vi "Main Single Channel Only.vi"() -> ()   [LabVIEW 2017]
uses:
  Controls/Timing Controls.ctl
  Controls/File Controls.ctl
  Controls/DAQ State.ctl
  <vilib>/DAQmx/write.llb/DAQmx Write (Analog 1D DBL NChan 1Samp).vi
  <vilib>/DAQmx/configure/timing.llb/DAQmx Timing (Sample Clock).vi
  <vilib>/DAQmx/miscellaneous.llb/DAQmx Fill In Error Info.vi
panel:
  in  "Trigger Channel (Find Using NI Max)":tag="Dev1/ai16"
  in  "Differential Value":dbl format="%#_13g"
  in  "Lower Limit":dbl=-0.85
  in  "Upper Limit":dbl=-0.75
  out "Differential":cluster{dbl[], dbl[]}[](graph)=[{[0.0, 1.0], [0.0029010882279960626, 0.00862868344710327]}, {[-1.0, 2.0], [-0.75, -0.75]}, {[-1.0, 2.0], [-0.85, -0.85]}]
  out "Saving?":bool
  out "Zero Values Dev1":dbl[](array[numeric])
  in  "Save":bool
  in  "File Control":T1={"File Path"=path "C:/Users/Force PC/Documents/Acquisition Data", "File Name"=""}
  out "Trigger":dynamicdata(graph)=[{"t0"=timestamp(3616576961.7901273 s since 1904-01-01), "dt"=0.001, "Y"=[2.8935987566836108, 2.892940411376444, 2.8932695840305964, 2.8932695840305964, 2.8932695840305964, 2.8932695840305964, 2.8934341703572457, 2.8935987566836108, 2.8935987566836108, 2.893763343009691, 2.8934341703572457, 2.8940925156609985, 2.8940925156609985, 2.8942571019862253, 2.8940925156609985, 2.8935987566836108, 2.893927929335487, 2.893763343009691, 2.893763343009691, 2.8934341703572457, 2.8932695840305964, 2.8932695840305964, 2.8931049977036625, 2.8934341703572457, 2.8931049977036625, 2.8932695840305964, 2.8931049977036625, 2.8935987566836108, 2.893927929335487, 2.893927929335487, 2.893763343009691, 2.8942571019862253, 2.8942571019862253, 2.8940925156609985, 2.893927929335487, 2.893927929335487, 2.893763343009691, 2.893763343009691, 2.8935987566836108, 2.8932695840305964, 2.8934341703572457, 2.892775825048941, 2.8931049977036625, 2.892940411376444, 2.8931049977036625, 2.8934341703572457, 2.8934341703572457, 2.893763343009691, 2.893763343009691, 2.893927929335487, 2.893763343009691, 2.894421688311168, 2.8942571019862253, 2.894421688311168, 2.8940925156609985, 2.893927929335487, 2.894421688311168, 2.894421688311168, 2.893763343009691, 2.8934341703572457, 2.893927929335487, 2.892940411376444, 2.8935987566836108, 2.8931049977036625, 2.8934341703572457, 2.8935987566836108, 2.8935987566836108, 2.893763343009691, 2.893763343009691, 2.8942571019862253, 2.893927929335487, 2.894421688311168, 2.8947508609601993, 2.894421688311168, 2.8940925156609985, 2.8940925156609985, 2.8942571019862253, 2.8940925156609985, 2.893763343009691, 2.8935987566836108, 2.8934341703572457, 2.8931049977036625, 2.892940411376444, 2.8931049977036625, 2.8932695840305964, 2.8931049977036625, 2.8932695840305964, 2.8935987566836108, 2.8935987566836108, 2.8942571019862253, 2.893927929335487, 2.894421688311168, 2.893927929335487, 2.894586274635826, 2.893927929335487, 2.8942571019862253, 2.893927929335487, 2.8940925156609985, 2.893763343009691, 2.8932695840305964], "attributes"=variant("NI_ChannelName"=variant(string "Trigger"), "NI_UnitDescription"=variant(string "Volts"))}]
  out "Dev1":dynamicdata(graph)=[{"t0"=timestamp(3616576961.790079 s since 1904-01-01), "dt"=0.001, "Y"=[0.004713341620051992, 0.0045485913126213084, 0.005042842234350253, 0.0052075925412182755, 0.004219090697197281, 0.0038895900810222983, 0.004219090697197281, 0.0043838410050032195, 0.0038895900810222983, 0.0037248397726536986, 0.004713341620051992, 0.0045485913126213084, 0.0045485913126213084, 0.004054340389203492, 0.0038895900810222983, 0.004713341620051992, 0.004713341620051992, 0.003395339155353394, 0.004878091927295269, 0.004219090697197281, 0.0038895900810222983, 0.003395339155353394, 0.004219090697197281, 0.004713341620051992, 0.0030658385373025787, 0.003395339155353394, 0.0038895900810222983, 0.003395339155353394, 0.0038895900810222983, 0.003230588846421689, 0.003560089464097249, 0.003230588846421689, 0.002571587608819481, 0.003230588846421689, 0.0029010882279960626, 0.0037248397726536986, 0.0030658385373025787, 0.0037248397726536986, 0.0037248397726536986, 0.003560089464097249, 0.003230588846421689, 0.0037248397726536986, 0.003230588846421689, 0.0027363379185016967, 0.0027363379185016967, 0.002571587608819481, 0.003230588846421689, 0.003560089464097249, 0.0037248397726536986, 0.0029010882279960626, 0.0037248397726536986, 0.003395339155353394, 0.003560089464097249, 0.003395339155353394, 0.0038895900810222983, 0.0029010882279960626, 0.003230588846421689, 0.0030658385373025787, 0.0027363379185016967, 0.003395339155353394, 0.0030658385373025787, 0.004054340389203492, 0.003560089464097249, 0.0037248397726536986, 0.0029010882279960626, 0.003230588846421689, 0.002571587608819481, 0.0027363379185016967, 0.0030658385373025787, 0.004054340389203492, 0.0027363379185016967, 0.00240683729894986, 0.002571587608819481, 0.0019125863682161182, 0.0027363379185016967, 0.0029010882279960626, 0.0030658385373025787, 0.0027363379185016967, 0.0030658385373025787, 0.0029010882279960626, 0.00240683729894986, 0.0030658385373025787, 0.0027363379185016967, 0.00240683729894986, 0.002571587608819481, 0.0030658385373025787, 0.003230588846421689, 0.002571587608819481, 0.002242086988892833, 0.003230588846421689, 0.002242086988892833, 0.002242086988892833, 0.0030658385373025787, 0.002571587608819481, 0.003230588846421689, 0.002571587608819481, 0.00240683729894986, 0.004054340389203492, 0.0029010882279960626, 0.0029010882279960626], "attributes"=variant("NI_ChannelName"=variant(string "Dev1_Ch3"), "NI_UnitDescription"=variant(string "Volts"))}]
  in  "Zero Dev1":bool caption="Zero"
  in  "Timing":T2={"Sampling Rate (Hz)"=1000.0, "Display Rate (Hz)"=100.0, "Sampling Mode"=10123} {"Sampling Mode" items=["Finite Samples"=10178, "Continuous Samples"=10123, "Hardware Timed Single Point"=12522]; "Sampling Rate (Hz)" format="%0.2f"}
  in  "Run":bool
  out "DAQ \nConnected?":bool
  in  "stop":bool
  # "You shouldn't need to change this,\nunless the trigger is not showing up.\nUse NI MAX -> Test Panels\nWill be between ai16 and ai31\nThis must be set before the program\nruns"
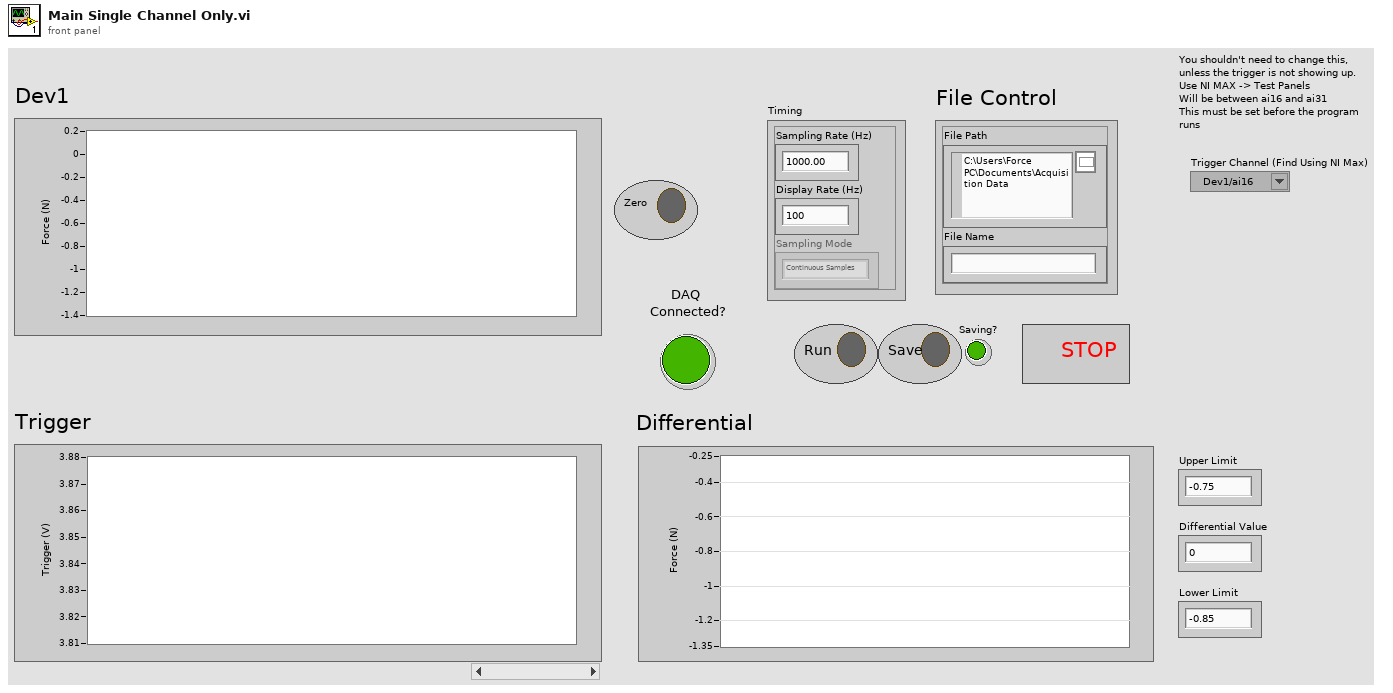
[diagram p1: front panel]
types:
  T1 = typedef "File Controls.ctl" = cluster{"File Path":path, "File Name":string}
  T2 = typedef "Timing Controls.ctl" = cluster{"Sampling Rate (Hz)":dbl, "Display Rate (Hz)":dbl, "Sampling Mode":i32}
  T3 = cluster{"Waveform Array":waveform(dbl)[][], bool}
  T4 = typedef "DAQ State.ctl" = enum16{"Init", "Wait", "Update Timing", "Zero Dev1", "Zero Dev2", "Start Task", "Read", "Stop Task", "Display Data", "Write to File", "Error Handling", "Shutdown"}
  T5 = enum8{"Enabled", "Disabled", "Disabled and Grayed Out"}
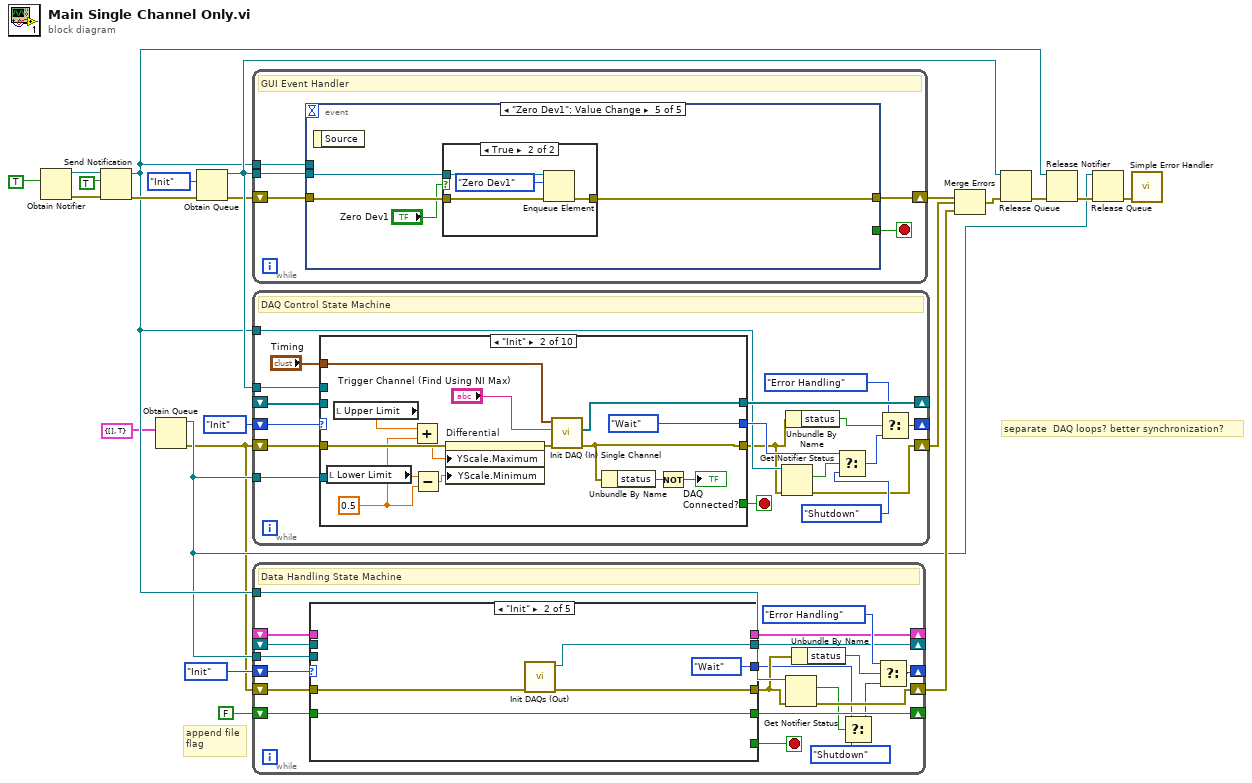
[diagram p0: block diagram]
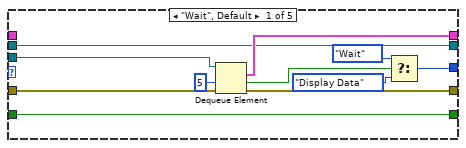
[diagram p2: hidden frame]
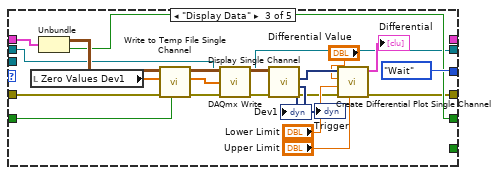
[diagram p3: hidden frame]
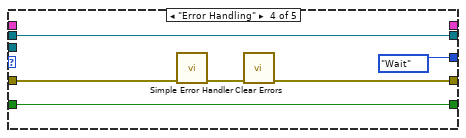
[diagram p4: hidden frame]
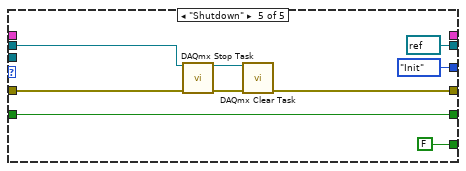
[diagram p5: hidden frame]
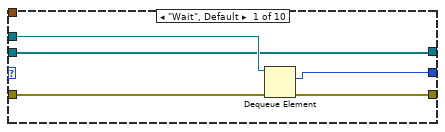
[diagram p6: hidden frame]
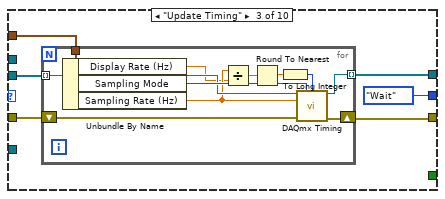
[diagram p7: hidden frame]
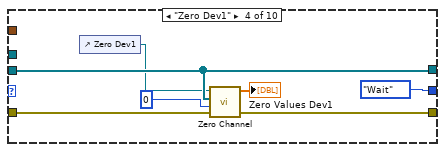
[diagram p8: hidden frame]
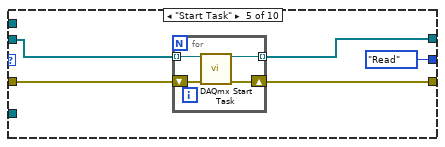
[diagram p9: hidden frame]
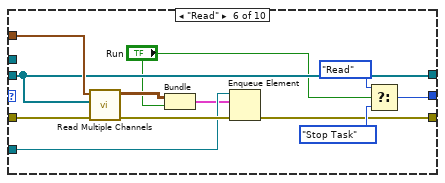
[diagram p10: hidden frame]
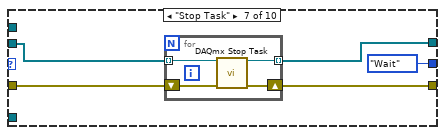
[diagram p11: hidden frame]
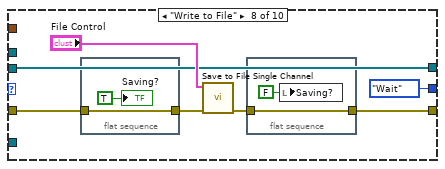
[diagram p12: hidden frame]
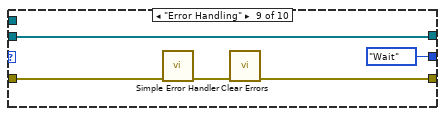
[diagram p13: hidden frame]
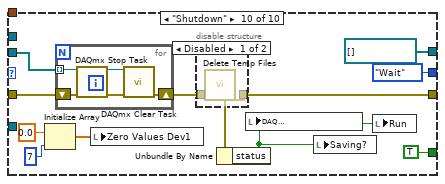
[diagram p14: hidden frame]
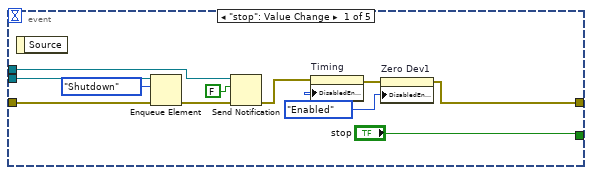
[diagram p16: hidden frame]
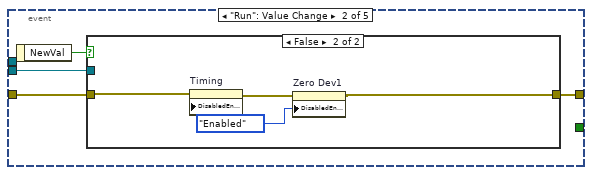
[diagram p17: hidden frame]
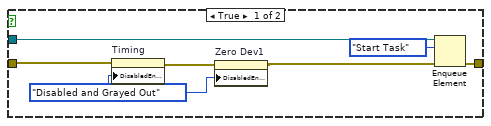
[diagram p18: hidden frame]
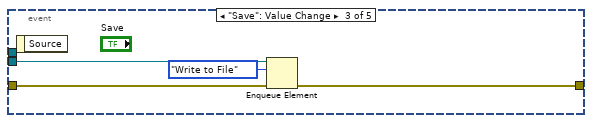
[diagram p19: hidden frame]
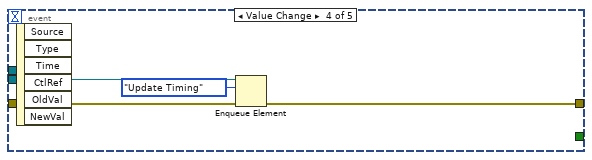
[diagram p20: hidden frame]
diagram:
  # "append file\nflag"
  # "separate  DAQ loops? better synchronization?"
  n1 = Obtain Notifier(notification data type=TRUE) -> (notifier out=w13:refnum<notifier>, error out=w12:errorcluster)  [unwired: 3 in, 1 out]
  n2 = Send Notification(notification=TRUE, notifier=w13, error in (no error)=w12) -> (notifier out=w9:refnum<notifier>, error out=w11:errorcluster)
  n3 = Obtain Queue(element data type=T3 {"Waveform Array"=[], TRUE}) -> (queue out=w6:refnum<queue>, error out=w2:errorcluster)  [unwired: 4 in, 1 out]
  n4 = Obtain Queue(element data type=DAQ_State."Init" ("DAQ State"), error in (no error)=w11) -> (queue out=w17:refnum<queue>, error out=w16:errorcluster)  [unwired: 3 in, 1 out]
  n5 = while {
    tunnel: w17 -> [w26]
    shift-right: [w24] -> w19
    shift-left: w16 -> [w25]
    tunnel: w9 -> [w23]
    stop <- w27 stop-if-true
    # "GUI Event Handler"
    n6 = event shown="[4] \"Zero Dev1\": Value Change" {
      selector: _ -> [_ _ _ _ _]
      dyn-events: _ -> [_ _ _ _ _]
      timeout: _ -> [_ _ _ _ _]
      tunnel: ["stop" _ _ _ _] -> w27
      tunnel: w26 -> [w36 w40 w55 w59 w63]
      tunnel: w25 -> [w37 w42 w57 w60 w64]
      tunnel: [w28 w41 w56 w61 w65] -> w24
      tunnel: w23 -> [w33 _ _ _ _]
      event "stop": Value Change {
        w30 = T5."Enabled" ("Disabled")
        n7 = event-data() -> ()  [unwired: 1 in, 1 out]
        n8 = Enqueue Element(queue=w36, element=DAQ_State."Shutdown", error in (no error)=w37) -> (error out=w34:errorcluster)  [unwired: 1 in, 2 out]
        n9 = Send Notification(notification=FALSE, notifier=w33, error in (no error)=w34) -> (error out=w29:errorcluster)  [unwired: 1 out]
        n10 = property on="Timing" class="Clust (strict)"(error in=w29, "DisabledEnum"=w30) -> (error out=w31:errorcluster)  [unwired: 1 in, 1 out]
        n11 = property on="Zero Dev1" class="Bool (strict)"(error in=w31, "DisabledEnum"=w30) -> (error out=w28:errorcluster)  [unwired: 1 in, 1 out]
      }
      event "Run": Value Change {
        n12 = event-data() -> ("NewVal"=w39:bool)  [unwired: 1 in]
        n13 = case shown="False" w39 {
          tunnel: w42 -> [w46 w53]
          tunnel: [w49 w50] -> w41
          tunnel: w40 -> [w48 _]
          frame True {
            w44 = T5."Disabled and Grayed Out" ("Disabled")
            n14 = property on="Timing" class="Clust (strict)"(error in=w46, "DisabledEnum"=w44) -> (error out=w45:errorcluster)  [unwired: 1 in, 1 out]
            n15 = property on="Zero Dev1" class="Bool (strict)"(error in=w45, "DisabledEnum"=w44) -> (error out=w43:errorcluster)  [unwired: 1 in, 1 out]
            n16 = Enqueue Element(queue=w48, element=DAQ_State."Start Task", error in (no error)=w43) -> (error out=w49:errorcluster)  [unwired: 1 in, 2 out]
          }
          frame False {
            w51 = T5."Enabled" ("Disabled")
            n17 = property on="Timing" class="Clust (strict)"(error in=w53, "DisabledEnum"=w51) -> (error out=w52:errorcluster)  [unwired: 1 in, 1 out]
            n18 = property on="Zero Dev1" class="Bool (strict)"(error in=w52, "DisabledEnum"=w51) -> (error out=w50:errorcluster)  [unwired: 1 in, 1 out]
          }
        }
      }
      event "Save": Value Change {
        n19 = event-data() -> ()  [unwired: 1 in, 1 out]
        n20 = Enqueue Element(queue=w55, element=DAQ_State."Write to File", error in (no error)=w57) -> (error out=w56:errorcluster)  [unwired: 1 in, 2 out]
      }
      event Value Change {
        n21 = event-data() -> ()  [unwired: 1 in, 6 out]
        n22 = Enqueue Element(queue=w59, element=DAQ_State."Update Timing", error in (no error)=w60) -> (error out=w61:errorcluster)  [unwired: 1 in, 2 out]
      }
      event "Zero Dev1": Value Change {
        n23 = event-data() -> ()  [unwired: 1 in, 1 out]
        n24 = case shown="True" "Zero Dev1" {
          tunnel: [w66 w69] -> w65
          tunnel: w64 -> [w66 w68]
          tunnel: w63 -> [_ w67]
          frame False {
          }
          frame True {
            n25 = Enqueue Element(queue=w67, element=DAQ_State."Zero Dev1", error in (no error)=w68) -> (error out=w69:errorcluster)  [unwired: 1 in, 2 out]
          }
        }
      }
    }
  }
  n26 = while {
    shift-right: [w81] -> _
    shift-left: DAQ_State."Init" ("DAQ State") -> [w88]
    shift-right: [w72] -> w20
    shift-left: w2 -> [w87]
    tunnel: w17 -> [w85]
    shift-right: [w84] -> _
    shift-left: _ -> [w83]
    tunnel: w6 -> [w75]
    tunnel: w9 -> [w74]
    stop <- w86 stop-if-true
    # "DAQ Control State Machine"
    n27 = case shown="\"Init\"" w88 {
      tunnel: [w90 DAQ_State."Wait" ("DAQ State") DAQ_State."Wait" ("DAQ State") DAQ_State."Wait" ("DAQ State") DAQ_State."Read" ("DAQ State") w150 DAQ_State."Wait" ("DAQ State") DAQ_State."Wait" ("DAQ State") DAQ_State."Wait" ("DAQ State") DAQ_State."Wait" ("DAQ State")] -> w78
      tunnel: [w93 w95 w112 w130 w135 w144 w156 w164 w176 w178] -> w73
      tunnel: w87 -> [w92 w102 w113 w131 w136 w152 w153 w163 w177 w187]
      tunnel: [_ _ _ _ _ _ _ _ _ TRUE] -> w86
      tunnel: w85 -> [w91 _ _ _ _ _ _ _ _ _]
      tunnel: [w89 w103 w108 w129 w133 w147 w157 w166 w173 refnum<k21>[] [] ("Channel Array")] -> w84
      tunnel: w83 -> [w89 _ w109 w129 w134 w147 w154 w166 w173 w185]
      tunnel: "Timing" -> [_ w104 w110 _ _ w148 _ _ _ _]
      tunnel: w75 -> [_ _ _ _ _ w145 _ _ _ _]
      frame "Wait", Default {
        n28 = Dequeue Element(queue=w91, error in (no error)=w92) -> (element=w90:T4, error out=w93:errorcluster)  [unwired: 1 in, 2 out]
      }
      frame "Init" {
        w97 = 0.5 ("Y Scale.Range:Maximum")
        n29 = local read "Lower Limit"() -> (w100:dbl)
        n30 = local read "Upper Limit"() -> (w98:dbl)
        n31 = Add(x=w98, y=w97) -> (x+y=w96:dbl)
        n32 = Subtract(x=w100, y=w97) -> (x-y=w99:dbl)
        n33 = property on="Differential" class="XYGraph (strict)"(error in=w102, "YScale.Maximum"=w96, "YScale.Minimum"=w99) -> (error out=w101:errorcluster)  [unwired: 1 in, 1 out]
        n34 = call "Init DAQ (In) Single Channel.vi"("error in (no error)"=w101, "Trigger Channel (Find Using NI Max)"="Trigger Channel (Find Using NI Max)", "Timing"=w104) -> ("error out"=w95:errorcluster, "Channel Array"=w103:refnum<k21>[])  [unwired: 7 in]
        n35 = Unbundle By Name(w95) -> ("status"=w106:bool)
        n36 = Not(x=w106) -> (.not. x?=→"DAQ \nConnected?":bool)
      }
      frame "Update Timing" {
        n37 = for {
          shift-right: [w123] -> w112
          shift-left: w113 -> [w124]
          tunnel: [w122] -> w108 mode=indexing
          tunnel: w110 -> [w121]
          tunnel: w109 -> [w119] mode=indexing
          n38 = Unbundle By Name(w121) -> ("Display Rate (Hz)"=w115:dbl, "Sampling Mode"=w120:i32, "Sampling Rate (Hz)"=w116:dbl)
          n39 = Divide(x=w116, y=w115) -> (x/y=w118:dbl)
          n40 = Round To Nearest(number=w118) -> (nearest integer value=w117:dbl)
          n41 = To Long Integer(number=w117) -> (32bit integer=w114:i32)
          n42 = call-poly <vilib>:"DAQmx Timing.vi"("task/channels in"=w119, "sample mode"=w120, "samples per channel"=w114, "rate"=w116, "error in"=w124) -> ("task out"=w122:refnum<k21>, "error out"=w123:errorcluster)  [unwired: 9 in]
        }
      }
      frame "Zero Dev1" {
        n43 = control-ref of="Zero Dev1"() -> (w127:refnum<vi>)
        n44 = call "Zero Channel.vi"("error in (no error)"=w131, "Dev to Zero"=0, "Channel Array"=w129, "Refnum"=w127) -> ("error out"=w130:errorcluster, "Zero Values"=→"Zero Values Dev1":dbl[])  [unwired: 6 in]
      }
      frame "Start Task" {
        n45 = for {
          shift-right: [w139] -> w135
          shift-left: w136 -> [w140]
          tunnel: w134 -> [w138] mode=indexing
          tunnel: [w137] -> w133 mode=indexing
          n46 = call <vilib>:"DAQmx Start Task.vi"("task/channels in"=w138, "error in"=w140) -> ("task out"=w137:refnum<k21>, "error out"=w139:errorcluster)  [unwired: 12 in]
        }
      }
      frame "Read" {
        n47 = call "Read Multiple Channels.vi"("error in (no error)"=w152, "Channel Array"=w147, "Timing"=w148) -> ("error out"=w146:errorcluster, "data"=w142:waveform(dbl)[][])  [unwired: 7 in]
        n48 = Bundle("data"=w142, "Run"="Run") -> (w143:cluster{"data":waveform(dbl)[][], "Run":bool})  [unwired: 1 in]
        n49 = Enqueue Element(queue=w145, element=w143, error in (no error)=w146) -> (error out=w144:errorcluster)  [unwired: 1 in, 2 out]
        n50 = Select(t=DAQ_State."Read", s="Run", f=DAQ_State."Stop Task" ("DAQ State")) -> (s? t:f=w150:T4)
      }
      frame "Stop Task" {
        n51 = for {
          shift-right: [w159] -> w156
          shift-left: w153 -> [w160]
          tunnel: w154 -> [w161] mode=indexing
          tunnel: [w158] -> w157 mode=indexing
          n52 = call <vilib>:"DAQmx Stop Task.vi"("task/channels in"=w161, "error in"=w160) -> ("task out"=w158:refnum<k21>, "error out"=w159:errorcluster)  [unwired: 12 in]
        }
      }
      frame "Write to File" {
        n53 = flat-sequence {
          tunnel: w163 -> [w170]
          tunnel: [w170] -> w162
          frame #0 {
            "Saving?" <- TRUE ("Saving?")
          }
        }
        n54 = call "Save to File Single Channel.vi"("error in (no error)"=w162, "File Control"="File Control") -> ("error out"=w165:errorcluster)  [unwired: 9 in]
        n55 = flat-sequence {
          tunnel: w165 -> [w172]
          tunnel: [w172] -> w164
          frame #0 {
            n56 = local write "Saving?"(FALSE ("Saving?")) -> ()
          }
        }
      }
      frame "Error Handling" {
        n57 = call <vilib>:"Simple Error Handler.vi"("error in (no error)"=w177) -> ("error out"=w175:errorcluster)  [unwired: 4 in, 4 out]
        n58 = call <vilib>:"Clear Errors.vi"("error in (no error)"=w175) -> ("error out"=w176:errorcluster)  [unwired: 5 in, 1 out]
      }
      frame "Shutdown" {
        n59 = Initialize Array(0.0 ("element"), 7 ("dimension size")) -> (w182:dbl[])
        n60 = for {
          shift-right: [w196] -> w183
          shift-left: w187 -> [w193]
          tunnel: w185 -> [w195] mode=indexing
          n61 = call <vilib>:"DAQmx Stop Task.vi"("task/channels in"=w195, "error in"=w193) -> ("task out"=w194:refnum<k21>, "error out"=w192:errorcluster)  [unwired: 12 in]
          n62 = call <vilib>:"DAQmx Clear Task.vi"("task in"=w194, "error in"=w192) -> ("error out"=w196:errorcluster)  [unwired: 13 in]
        }
        n63 = local write "Zero Values Dev1"(w182) -> ()
        n64 = disable-structure shown="Disabled" {
          disable-tunnel: w183 -> [w190 w191]
          disable-tunnel: [w189 w191] -> w178
          frame Disabled {
            n65 = call "Delete Temp Files.vi"("error in (no error)"=w190) -> ("error out"=w189:errorcluster)  [unwired: 10 in]
          }
          frame Enabled {
          }
        }
        n66 = Unbundle By Name(w183) -> ("status"=w179:bool)
        n67 = local write "DAQ \nConnected?"(w179) -> ()
        n68 = local write "Saving?"(w179) -> ()
        n69 = local write "Run"(w179) -> ()
      }
    }
    n70 = Get Notifier Status(notifier=w74, error in (no error)=w73) -> (current notification=w71:bool, error out=w72:errorcluster)  [unwired: 3 out]
    n71 = Unbundle By Name(w73) -> ("status"=w82:bool)
    n72 = Select(t=w78, s=w71, f=DAQ_State."Shutdown" ("t")) -> (s? t:f=w77:T4)
    n73 = Select(t=DAQ_State."Error Handling", s=w82, f=w77) -> (s? t:f=w81:T4)
  }
  n74 = while {
    shift-right: [w206] -> _
    shift-left: DAQ_State."Init" ("DAQ State") -> [w216]
    shift-right: [w209] -> w7
    shift-left: w2 -> [w215]
    tunnel: w9 -> [w214]
    tunnel: w6 -> [w213]
    shift-right: [w208] -> _
    shift-left: _ -> [w207]
    shift-right: [w204] -> _
    shift-left: FALSE ("Append to file?") -> [w205]
    shift-right: [w198] -> _
    shift-left: _ -> [w197]
    stop <- w203 stop-if-true
    # "Data Handling State Machine"
    n75 = case shown="\"Init\"" w216 {
      tunnel: w215 -> [w227 w232 w251 w258 w260]
      tunnel: [w226 w230 w239 w257 w267] -> w210
      tunnel: w213 -> [w225 _ _ _ _]
      tunnel: [w219 DAQ_State."Wait" ("t") DAQ_State."Wait" ("t") DAQ_State."Wait" ("t") DAQ_State."Init" ("t")] -> w201
      tunnel: [w224 _ _ _ _] -> w208
      tunnel: w207 -> [_ _ w250 _ _]
      tunnel: w205 -> [w218 w228 w246 w255 w262]
      tunnel: [w218 w228 w248 w255 w262] -> w204
      tunnel: [_ _ _ _ FALSE] -> w203
      tunnel: [w217 w231 w233 w254 refnum<k21> refnum ("Channel")] -> w198
      tunnel: w197 -> [w217 _ w234 w254 w261]
      frame "Wait", Default {
        n76 = Dequeue Element(queue=w225, timeout in ms (-1)=5, error in (no error)=w227) -> (element=w224:T3, timed out?=w222:bool, error out=w226:errorcluster)  [unwired: 1 out]
        n77 = Select(t=DAQ_State."Wait", s=w222, f=DAQ_State."Display Data" ("t")) -> (s? t:f=w219:T4)
      }
      frame "Init" {
        n78 = call "Init DAQs (Out).vi"("error in (no error)"=w232) -> ("error out"=w230:errorcluster, "Channel"=w231:refnum<k21>)  [unwired: 9 in]
      }
      frame "Display Data" {
        n79 = local read "Zero Values Dev1"() -> (w247:dbl[])
        n80 = Unbundle(w250) -> ("Waveform Array"=w249:waveform(dbl)[][], w248:bool)
        n81 = call "Write to Temp File Single Channel.vi"("Append to file?"=w246, "error in (no error)"=w251, "Dev1 Zero Values"=w247, "Waveform Array"=w249) -> ("error out"=w236:errorcluster, "Fx and Fy"=w237:dbl[], "Zeroed Array"=w245:waveform(dbl)[][])  [unwired: 5 in]
        n82 = call-poly <vilib>:"DAQmx Write.vi"("task/channels in"=w234, "data"=w237, "error in"=w236) -> ("task out"=w233:refnum<k21>, "error out"=w235:errorcluster)  [unwired: 10 in, 1 out]
        n83 = call "Display Single Channel.vi"("Error In"=w235, "Waveform Array"=w245) -> ("Error Out"=w240:errorcluster, "Trigger"=→"Trigger":dynamicdata, "Dev1 Ch3"=w244:dynamicdata)  [unwired: 7 in]
        "Dev1" <- w244
        n84 = call "Create Differential Plot Single Channel.vi"("Upper Limit"="Upper Limit", "Error In"=w240, "Lower Limit"="Lower Limit", "Differential Value"="Differential Value", "Dev1 Ch3"=w244) -> ("Error Out"=w239:errorcluster, "Array"=→"Differential":cluster{"Array":dbl[], "Array":dbl[]}[])  [unwired: 5 in]
      }
      frame "Error Handling" {
        n85 = call <vilib>:"Simple Error Handler.vi"("error in (no error)"=w258) -> ("error out"=w259:errorcluster)  [unwired: 4 in, 4 out]
        n86 = call <vilib>:"Clear Errors.vi"("error in (no error)"=w259) -> ("error out"=w257:errorcluster)  [unwired: 5 in, 1 out]
      }
      frame "Shutdown" {
        n87 = call <vilib>:"DAQmx Stop Task.vi"("task/channels in"=w261, "error in"=w260) -> ("task out"=w265:refnum<k21>, "error out"=w266:errorcluster)  [unwired: 12 in]
        n88 = call <vilib>:"DAQmx Clear Task.vi"("task in"=w265, "error in"=w266) -> ("error out"=w267:errorcluster)  [unwired: 13 in]
      }
    }
    n89 = Get Notifier Status(notifier=w214, error in (no error)=w210) -> (current notification=w202:bool, error out=w209:errorcluster)  [unwired: 3 out]
    n90 = Unbundle By Name(w210) -> ("status"=w211:bool)
    n91 = Select(t=w201, s=w202, f=DAQ_State."Shutdown") -> (s? t:f=w200:T4)
    n92 = Select(t=DAQ_State."Error Handling", s=w211, f=w200) -> (s? t:f=w206:T4)
  }
  n93 = Merge Errors(w19, w20, w7) -> (w18:errorcluster)
  n94 = Release Queue(queue=w17, error in (no error)=w18) -> (error out=w1:errorcluster)  [unwired: 1 in, 2 out]
  n95 = Release Notifier(notifier=w9, error in (no error)=w1) -> (error out=w8:errorcluster)  [unwired: 1 in, 2 out]
  n96 = Release Queue(queue=w6, error in (no error)=w8) -> (error out=w5:errorcluster)  [unwired: 1 in, 2 out]
  n97 = call <vilib>:"Simple Error Handler.vi"("error in (no error)"=w5) -> ()  [unwired: 4 in, 5 out]
